vi "Handle SUBSCRIBED.vi"(0 "reference":refnum<class "WAMP Client.lvclass">, 5 "error in (no error)":errorcluster, 7 "WAMP Message":T1 {"Message Codes" items=["HELLO"=1, "WELCOME"=2, "ABORT"=3, "GOODBYE"=6, "ERROR"=8, "PUBLISH"=16, "PUBLISHED"=17, "SUBSCRIBE"=32, "SUBSCRIBED"=33, "UNSUBSCRIBE"=34, "UNSUBSCRIBED"=35, "EVENT"=36, "CALL"=48, "RESULT"=59, "REGISTER"=64, "REGISTERED"=65, "UNREGISTER"=66, "UNREGISTERED"=67, "INVOCATION"=68, "YIELD"=70]}, 9 "Subscription Requests In":map{u32, T4}(c390), 11 "Subscriptions In":map{u32, T3}(c390)) -> (4 "reference out":refnum<class "WAMP Client.lvclass">, 6 "error out":errorcluster, 10 "Subscription Requests Out":map{u32, T4}(c390), 15 "Subscriptions Map Out":map{u32, T3}(c390))   [LabVIEW 2020, in "WAMP Client.lvclass"]
uses:
  <userlib>/wamplv/WAMP Client/WAMP Client.lvclass
  <userlib>/wamplv/WAMP Client/TypeDef/SUBSCRIBE Request Data.ctl
  <userlib>/wamplv/WAMP Client/TypeDef/Subscribe Result.ctl
  <userlib>/wamplv/WAMP Client/TypeDef/Event Payload.ctl
  <userlib>/wamplv/WAMP Client/TypeDef/Subscription Details.ctl
  <userlib>/wamplv/WAMP Client/TypeDef/WAMP Received Message.ctl
  <userlib>/wamplv/WAMP Message Codes.ctl
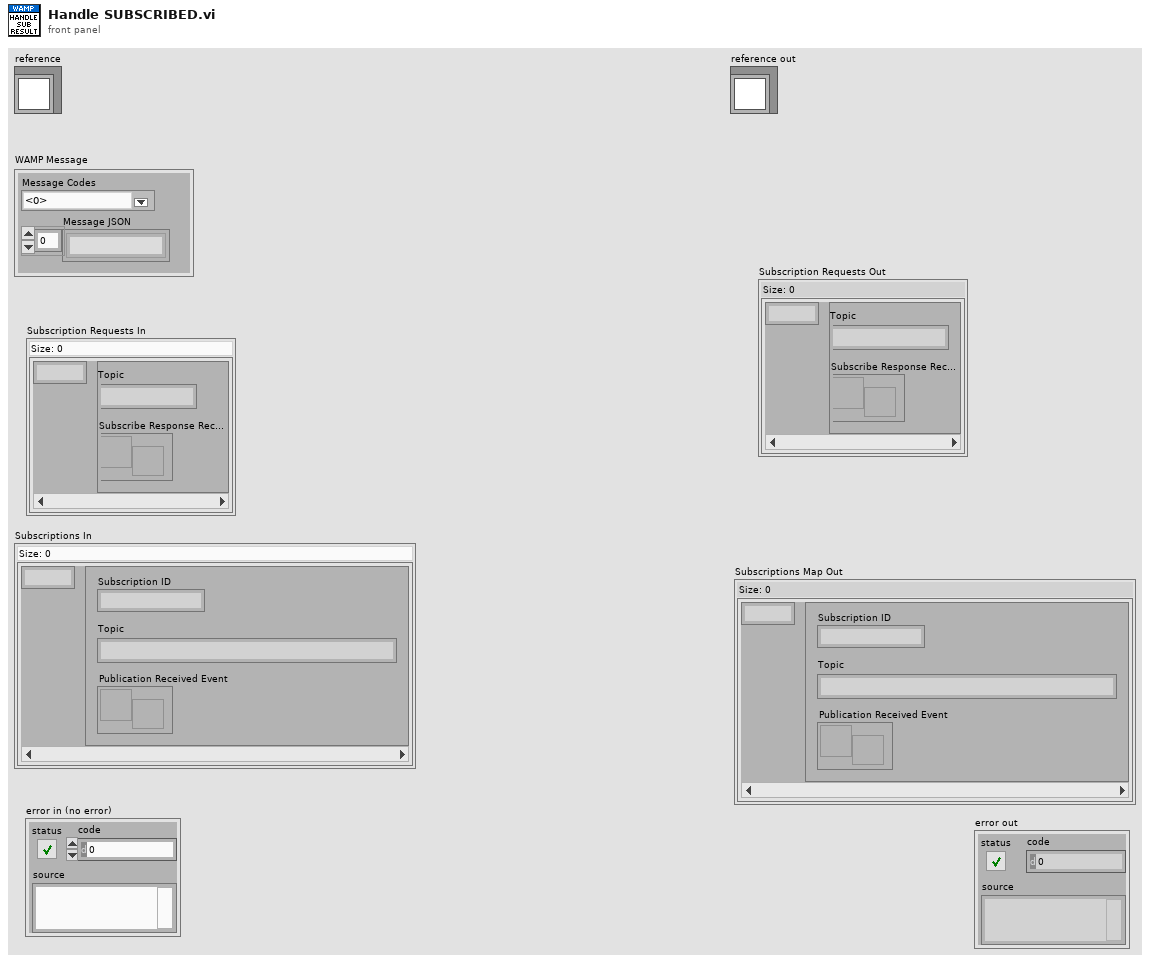
[diagram p1: front panel]
types:
  T1 = typedef "WAMP Client.lvclass/WAMP Received Message.ctl" = cluster{"Message JSON":string[], "Message Codes":T2}
  T2 = typedef "WAMP Client.lvclass/WAMP Message Codes.ctl" = u16
  T3 = typedef "WAMP Client.lvclass/Subscription Details.ctl" = cluster{"Subscription ID":u32, "Topic":string, "Publication Received Event":refnum<user-event>}
  T4 = typedef "WAMP Client.lvclass/SUBSCRIBE Request Data.ctl" = cluster{"Topic":string, "Subscribe Response Received Event":refnum<user-event>}
  T5 = typedef "WAMP Client.lvclass/SUBSCRIBE Result.ctl" = cluster{"Success?":bool, "Error":errorcluster, "Publication Received Event":refnum<user-event>}
  T6 = typedef "WAMP Client.lvclass/EVENT Payload.ctl" = cluster{"Arguments Payload":string[], "ArgumentKw Payload":string, "Topic":string}
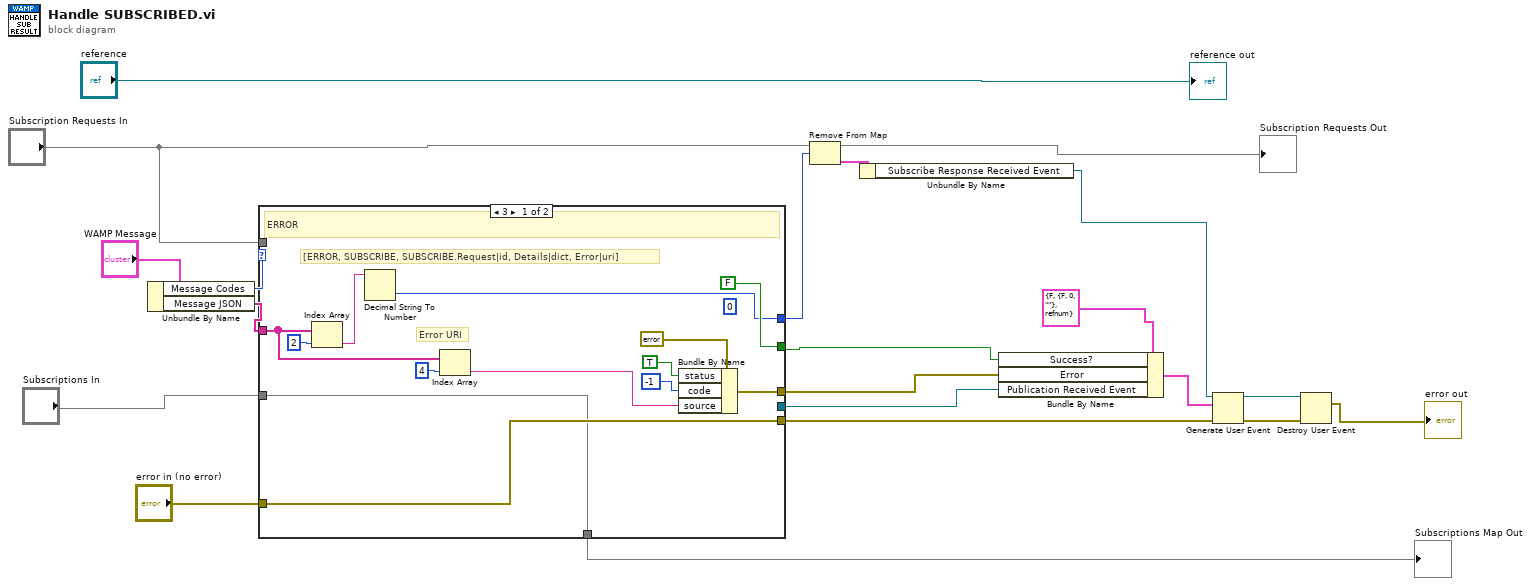
[diagram p0: block diagram]
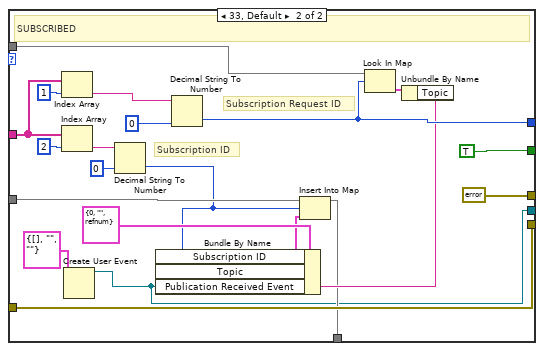
[diagram p2: hidden frame]
diagram:
  n1 = Unbundle By Name("WAMP Message") -> ("Message Codes"=w13:T2, "Message JSON"=w12:string[])
  n2 = case shown="3" w13 {
    tunnel: w12 -> [w32 w52]
    tunnel: [w23 w40] -> w11
    tunnel: "error in (no error)" -> [w26 w51]
    tunnel: [w26 w51] -> w16
    tunnel: [w27 errorcluster {"status"=FALSE, "code"=0, "source"=""} ("error in (no error)")] -> w19
    tunnel: [FALSE ("Success?") TRUE ("Success?")] -> w18
    tunnel: "Subscriptions In" -> [w22 w45]
    tunnel: "Subscription Requests In" -> [_ w41]
    tunnel: [w22 w36] -> w2
    tunnel: [_ w35] -> w1
    frame 3 {
      (unwired) 0
      # "Error URI"
      # "[ERROR, SUBSCRIBE, SUBSCRIBE.Request|id, Details|dict, Error|uri]"
      # "ERROR"
      n3 = Index Array(array=w32, index=2) -> (element=w33:string)
      n4 = Decimal String To Number(string=w33) -> (number=w23:i32)  [unwired: 2 in, 1 out]
      n5 = Index Array(array=w32, index=4) -> (element=w29:string)
      n6 = Bundle By Name(cluster=errorcluster {"status"=FALSE, "code"=0, "source"=""} ("error in (no error)"), "status"=TRUE, "code"=-1, "source"=w29) -> (w27:errorcluster)
    }
    frame 33, Default {
      # "Subscription Request ID"
      # "Subscription ID"
      # "SUBSCRIBED"
      n7 = Index Array(array=w52, index=1) -> (element=w48:string)
      n8 = Index Array(array=w52, index=2) -> (element=w54:string)
      n9 = Create User Event(user event datatype=T6 {"Arguments Payload"=[], "ArgumentKw Payload"="", "Topic"=""} ("Cluster")) -> (user event=w35:refnum<user-event>)  [unwired: 1 in, 1 out]
      n10 = Decimal String To Number(string=w54, default (0L)=u32 0) -> (number=w43:u32)  [unwired: 1 in, 1 out]
      n11 = Decimal String To Number(string=w48, default (0L)=u32 0) -> (number=w40:u32)  [unwired: 1 in, 1 out]
      n12 = Look In Map(map=w41, key=w40) -> (value=w39:T4)  [unwired: 1 in, 1 out]
      n13 = Unbundle By Name(w39) -> ("Topic"=w38:string)
      n14 = Bundle By Name(cluster=T3 {"Subscription ID"=0, "Topic"="", "Publication Received Event"=refnum} ("Cluster"), "Subscription ID"=w43, "Topic"=w38, "Publication Received Event"=w35) -> (w42:T3)
      n15 = Insert Into Map(map in=w45, key=w43, value=w42) -> (map out=w36:map{u32, T3})  [unwired: 2 out]
    }
  }
  "Subscriptions Map Out" <- w2
  n16 = Remove From Map(10:w11, 11:"Subscription Requests In") -> (1:w9:T4, 3:→"Subscription Requests Out":map{u32, T4})  [unwired: 1 out]
  n17 = Unbundle By Name(w9) -> ("Subscribe Response Received Event"=w8:refnum<user-event>)
  n18 = Bundle By Name(cluster=T5 {"Success?"=FALSE, "Error"={"status"=FALSE, "code"=0, "source"=""}, "Publication Received Event"=refnum} ("event data"), "Success?"=w18, "Error"=w19, "Publication Received Event"=w1) -> (w17:T5)
  n19 = Generate User Event(user event=w8, event data cluster=w17, error in=w16) -> (user event out=w5:refnum<user-event>, error out=w7:errorcluster)  [unwired: 1 in]
  n20 = Destroy User Event(user event=w5, error in=w7) -> (error out=→"error out":errorcluster)
  "reference out" <- "reference"
